vi "Calibratge.vi"() -> (0 "FuerzasCorte":string[](array[string]), 2 "Informe actiu 2":bool, 3 "OK ?":bool, 5 "Password 2":string, 6 "DeformacioOut":dbl caption="Deformació", 7 "VelocitatMaximaOut":dbl caption="Velocitat Máxima", 8 "VelocitatMotorOut":dbl caption="Velocitat Motor", 9 "Path 2":path)   [LabVIEW 2017]
uses:
  <vilib>/registry/registry.llb/Registry RtKey.ctl
  <vilib>/registry/registry.llb/Registry View.ctl
  <vilib>/registry/registry.llb/Write Registry Value Simple STR.vi
panel:
  in  "Path":path
  in  "Informe actiu":bool
  out "Informe":string
  in  "Password":string
  in  "VelocitatMaxima":dbl caption="Velocitat Máxima"
  in  "Table Control":string[][](table)
  in  "VelocitatMotor":dbl caption="Velocitat Motor"
  in  "Deformacio":dbl caption="Deformació"
  in  "error in (no error)":errorcluster
  in  "Cancel":bool
  in  "OK Button":bool
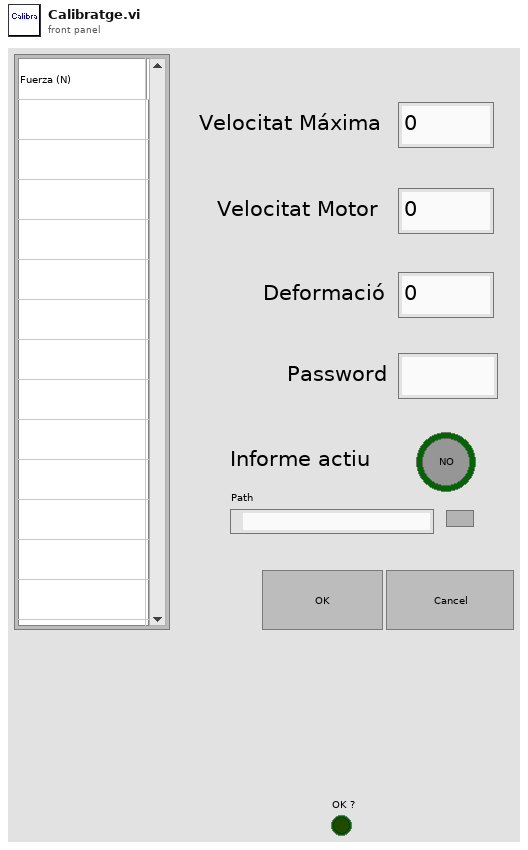
[diagram p1: front panel]
types:
  T1 = typedef "Registry RtKey.ctl" = enum32{"HKEY_CLASSES_ROOT", "HKEY_CURRENT_USER", "HKEY_LOCAL_MACHINE", "HKEY_USERS", "HKEY_PERFORMANCE_DATA", "HKEY_CURRENT_CONFIG", "HKEY_DYN_DATA"}
  T2 = typedef "Registry View.ctl" = u16
  T3 = typedef "Registry refnum.ctl" = refnum<k1>
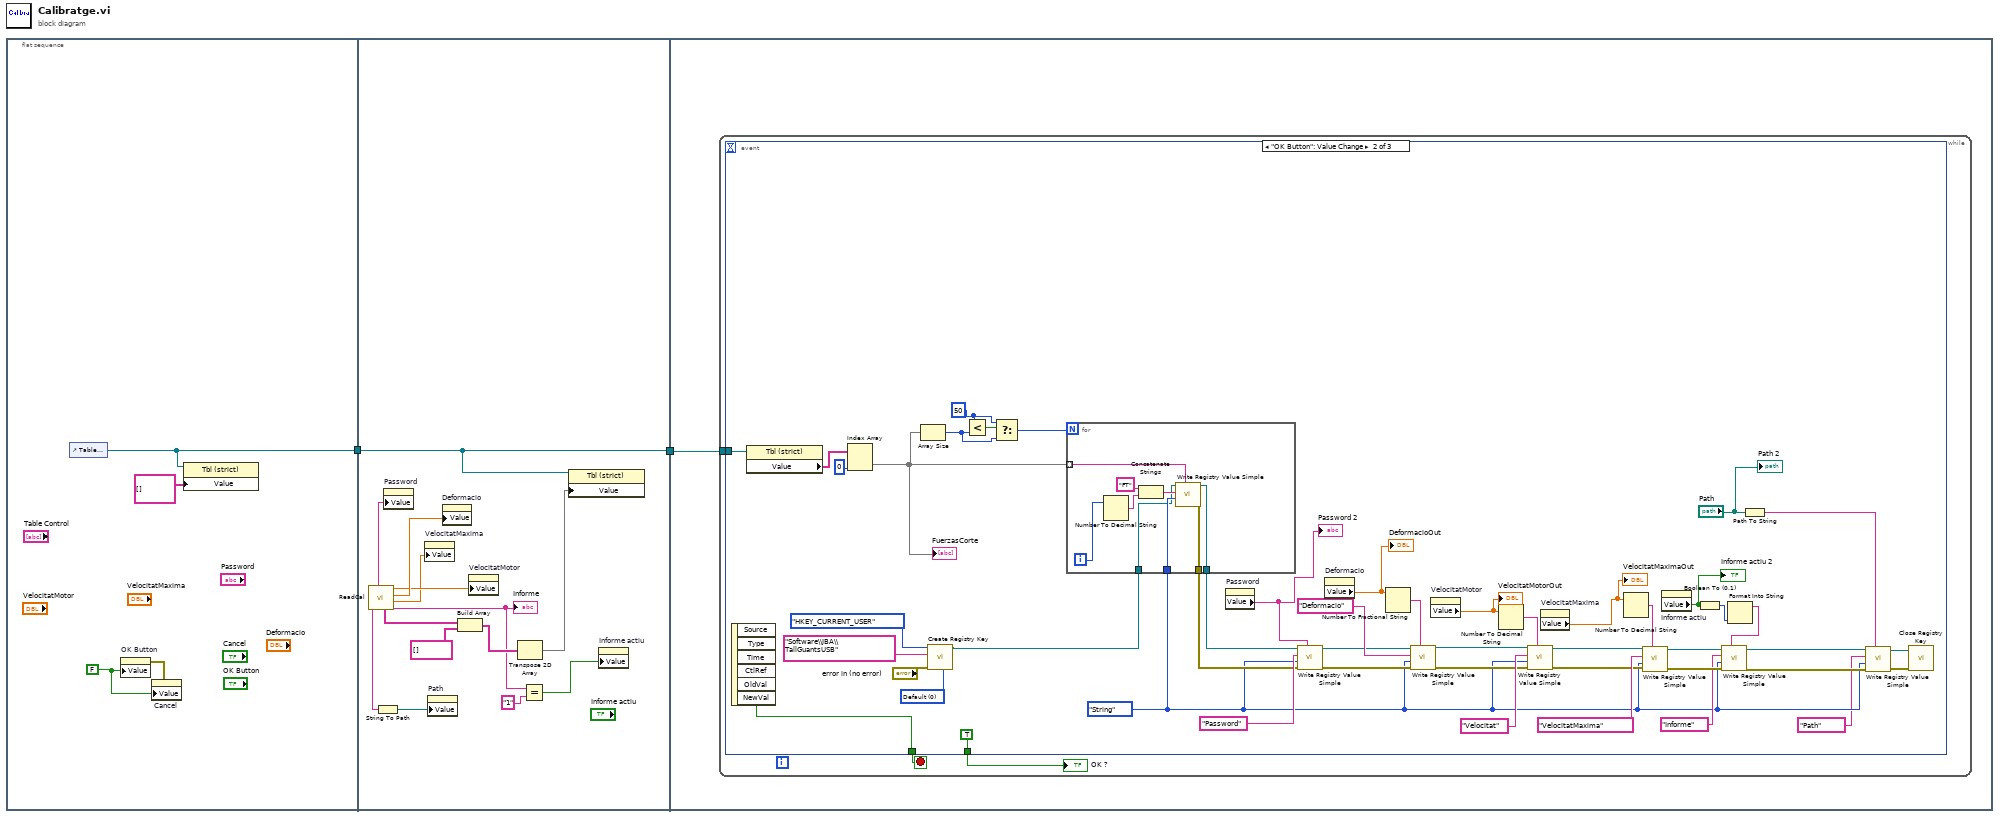
[diagram p0: block diagram]
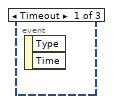
[diagram p2: hidden frame]
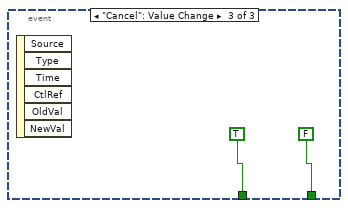
[diagram p3: hidden frame]
diagram:
  n1 = flat-sequence {
    tunnel: [w4] -> w1
    tunnel: [w20] -> w2
    tunnel: w1 -> [w20]
    tunnel: w2 -> [w21]
    frame #0 {
      w5 = FALSE ("OK Button")
      n2 = control-ref of="Table Control"() -> (w4:refnum<vi>)
      n3 = property on="OK Button" class="Bool (strict)"("Value"=w5) -> (error out=w6:errorcluster)  [unwired: 2 in, 1 out]
      n4 = property on="Cancel" class="Bool (strict)"(error in=w6, "Value"=w5) -> ()  [unwired: 1 in, 2 out]
      n5 = property class="Tbl (strict)"(reference=w4, "Value"=string[][] []) -> ()  [unwired: 1 in, 2 out]
    }
    frame #1 {
      n6 = call "ReadCal.vi"() -> ("Informe"=w11:string, "VelocitatMaxima"=w13:dbl, "Deformacio"=w19:dbl, "Velocitat"=w18:dbl, "Taula"=w17:string[], "Password"=w12:string, "Path"=w8:string)  [unwired: 3 in]
      "Informe" <- w11
      n7 = String To Path(string=w8) -> (path=w7:path)
      n8 = property on="Password" class="Str"("Value"=w12) -> ()  [unwired: 2 in, 2 out]
      n9 = property on="VelocitatMaxima" class="DigNum (strict)"("Value"=w13) -> ()  [unwired: 2 in, 2 out]
      n10 = property on="Path" class="Path"("Value"=w7) -> ()  [unwired: 2 in, 2 out]
      n11 = property on="Deformacio" class="DigNum (strict)"("Value"=w19) -> ()  [unwired: 2 in, 2 out]
      n12 = Build Array(w17, string[] [] ("element")) -> (w15:string[][])
      n13 = property on="VelocitatMotor" class="DigNum (strict)"("Value"=w18) -> ()  [unwired: 2 in, 2 out]
      n14 = Transpose 2D Array(2D array=w15) -> (transposed array=w14:string[][])
      n15 = Equal?(x=w11, y="1") -> (x = y?=w9:bool)
      n16 = property class="Tbl (strict)"(reference=w20, "Value"=w14) -> ()  [unwired: 1 in, 2 out]
      n17 = property on="Informe actiu" class="Bool (strict)"("Value"=w9) -> ()  [unwired: 2 in, 2 out]
    }
    frame #2 {
      n18 = while {
        tunnel: w21 -> [w22]
        stop <- w24 stop-if-true
        n19 = event shown="[1] \"OK Button\": Value Change" {
          selector: _ -> [_ _ _]
          dyn-events: _ -> [_ _ _]
          timeout: _ -> [_ _ _]
          tunnel: [_ w72 TRUE ("NewVal")] -> w24
          tunnel: [_ TRUE ("Ok?") FALSE ("Ok?")] -> w23
          tunnel: w22 -> [_ w59 _]
          event Timeout {
            n20 = event-data() -> ()  [unwired: 1 in, 2 out]
          }
          event "OK Button": Value Change {
            w58 = 50 ("y")
            w27 = enum16{"String", "Binary", "DWORD"}."String" ("simple data type")
            w64 = T2 0 items=["Default"=0, "KEY_WOW64_64KEY"=8, "KEY_WOW64_32KEY"=9] ("registry view")
            n21 = event-data() -> ("NewVal"=w72:bool)  [unwired: 1 in, 5 out]
            n22 = property class="Tbl (strict)"(reference=w59) -> ("Value"=w50:string[][])  [unwired: 1 in, 2 out]
            n23 = Index Array(array=w50, index (col)=0 ("disabled index (col)")) -> (element=w47:string[])  [unwired: 1 in]
            "FuerzasCorte" <- w47
            n24 = Array Size(array=w47) -> (size(s)=w56:i32)
            n25 = call <vilib>:"Create Registry Key.vi"("registry view"=w64, "error in (no error)"="error in (no error)", "subkey"="Software\\JBA\\TallGuantsUSB", "root key (HKEY_LOCAL_MACHINE)"=Registry_RtKey."HKEY_CURRENT_USER") -> ("refnum out"=w60:T3)  [unwired: 5 in, 2 out]
            n26 = Less?(x=w58, y=w56) -> (x < y?=w57:bool)
            n27 = Select(t=w58, s=w57, f=w56) -> (s? t:f=w55:i32)
            n28 = for {
              N: w55 -> [_]
              tunnel: w47 -> [w78] mode=indexing
              tunnel: w27 -> [w77]
              tunnel: w60 -> [w76]
              tunnel: [w75] -> w43
              tunnel: [w74] -> w42
              i -> [w81]
              n29 = Number To Decimal String(number=w81) -> (decimal integer string=w79:string)  [unwired: 1 in]
              n30 = Concatenate Strings("FT" ("value"), w79) -> (w80:string)
              n31 = call-poly <vilib>:"Write Registry Value Simple.vi"("String/Binary data"=w78, "simple data type"=w77, "value"=w80, "refnum"=w76) -> ("error out"=w74:errorcluster, "refnum out"=w75:T3)  [unwired: 4 in]
            }
            n32 = property on="Password" class="Str"() -> ("Value"=w41:string)  [unwired: 2 in, 2 out]
            "Password 2" <- w41
            n33 = call-poly <vilib>:"Write Registry Value Simple.vi"("String/Binary data"=w41, "error in (no error)"=w42, "simple data type"=w27, "value"="Password", "refnum"=w43) -> ("error out"=w45:errorcluster, "refnum out"=w46:T3)  [unwired: 3 in]
            n34 = property on="Deformacio" class="DigNum (strict)"() -> ("Value"=w34:dbl)  [unwired: 2 in, 2 out]
            "DeformacioOut" <- w34
            n35 = Number To Fractional String(number=w34) -> (F-format string=w33:string)  [unwired: 3 in]
            n36 = call-poly <vilib>:"Write Registry Value Simple.vi"("String/Binary data"=w33, "error in (no error)"=w45, "simple data type"=w27, "value"="Deformacio", "refnum"=w46) -> ("error out"=w61:errorcluster, "refnum out"=w62:T3)  [unwired: 3 in]
            n37 = property on="VelocitatMotor" class="DigNum (strict)"() -> ("Value"=w49:dbl)  [unwired: 2 in, 2 out]
            "VelocitatMotorOut" <- w49
            n38 = Number To Decimal String(number=w49) -> (decimal integer string=w68:string)  [unwired: 1 in]
            n39 = call-poly <vilib>:"Write Registry Value Simple.vi"("String/Binary data"=w68, "error in (no error)"=w61, "simple data type"=w27, "value"="Velocitat", "refnum"=w62) -> ("error out"=w52:errorcluster, "refnum out"=w51:T3)  [unwired: 3 in]
            n40 = property on="VelocitatMaxima" class="DigNum (strict)"() -> ("Value"=w48:dbl)  [unwired: 2 in, 2 out]
            "VelocitatMaximaOut" <- w48
            n41 = Number To Decimal String(number=w48) -> (decimal integer string=w53:string)  [unwired: 1 in]
            n42 = call-poly <vilib>:"Write Registry Value Simple.vi"("String/Binary data"=w53, "error in (no error)"=w52, "simple data type"=w27, "value"="VelocitatMaxima", "refnum"=w51) -> ("error out"=w40:errorcluster, "refnum out"=w39:T3)  [unwired: 3 in]
            n43 = property on="Informe actiu" class="Bool (strict)"() -> ("Value"=w35:bool)  [unwired: 2 in, 2 out]
            "Informe actiu 2" <- w35
            n44 = Boolean To (0,1)(Boolean=w35) -> (0, 1=w37:i16)
            n45 = Format Into String(w37) -> (resulting string=w36:string)  [unwired: 3 in, 1 out]
            n46 = call-poly <vilib>:"Write Registry Value Simple.vi"("String/Binary data"=w36, "error in (no error)"=w40, "simple data type"=w27, "value"="Informe", "refnum"=w39) -> ("error out"=w29:errorcluster, "refnum out"=w32:T3)  [unwired: 3 in]
            n47 = Path To String(path="Path") -> (string=w28:string)
            n48 = call-poly <vilib>:"Write Registry Value Simple.vi"("String/Binary data"=w28, "error in (no error)"=w29, "simple data type"=w27, "value"="Path", "refnum"=w32) -> ("error out"=w30:errorcluster, "refnum out"=w31:T3)  [unwired: 3 in]
            n49 = call <vilib>:"Close Registry Key.vi"("error in (no error)"=w30, "refnum"=w31) -> ()  [unwired: 5 in, 1 out]
            "Path 2" <- "Path"
          }
          event "Cancel": Value Change {
            n50 = event-data() -> ()  [unwired: 1 in, 6 out]
          }
        }
        "OK ?" <- w23
      }
    }
  }
